vi "test ping device.vi"() -> ()   [LabVIEW 2019]
panel:
  out "error out":errorcluster
  in  "error in":errorcluster
  in  "IP":string
  out "Active?":bool
  out "standard output":string
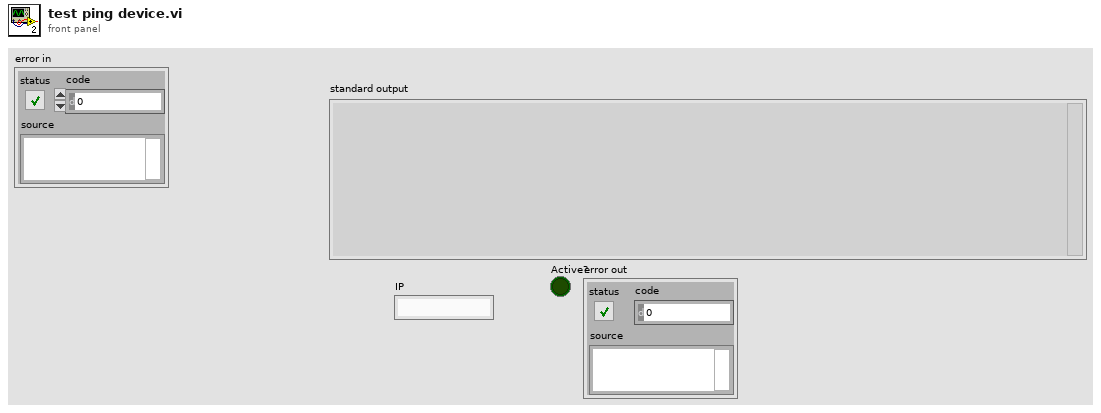
[diagram p1: front panel]
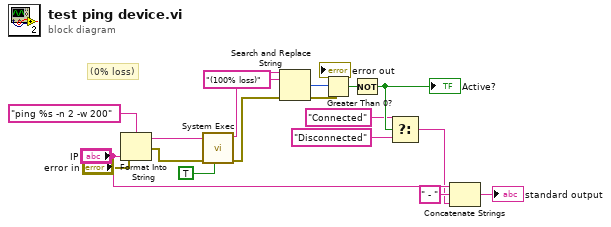
[diagram p0: block diagram]
diagram:
  # "(0% loss)"
  n1 = Format Into String(format string="ping %s -n 2 -w 200" ("command line"), error in="error in", "IP") -> (resulting string=w14:string, error out=w15:errorcluster)  [unwired: 1 in]
  n2 = call <vilib>:"System Exec.vi"("run minimized? (F)"=TRUE, "error in (no error)"=w15, "command line"=w14) -> ("error out"=w12:errorcluster, "standard output"=w7:string)  [unwired: 5 in, 2 out]
  n3 = Search and Replace String(input string=w7, search string="(100% loss)", error in=w12) -> (number of replacements=w11:i32, error out=→"error out":errorcluster)  [unwired: 5 in, 2 out]
  n4 = Greater Than 0?(x=w11) -> (x > 0?=w16:bool)
  n5 = Not(x=w16) -> (.not. x?=w6:bool)
  "Active?" <- w6
  n6 = Select(t="Connected" ("search string"), s=w6, f="Disconnected" ("search string")) -> (s? t:f=w4:string)
  n7 = Concatenate Strings("IP", " - " ("string"), w4) -> (→"standard output":string)
